vi "RSZVB Close.vi"(8 "error in (no error)":errorcluster {"code" format="%.0x"}, 11 "VISA session":refnum<visa-resource-name>) -> (0 "error out":errorcluster {"code" format="%.0x"})   [LabVIEW 2015]
doc: "This VI closes the I/O interface with the instrument."
uses:
  _utility/RSZVB Global Data.vi
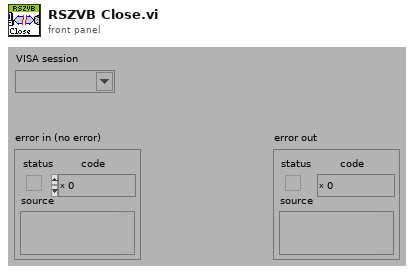
[diagram p1: front panel]
types:
  T1 = cluster{"Error Checking (T: On)":bool, "Installed Options":string[], "Data Valid?":bool, "Ports":i32, "Model":string[], "Option Checking (T: On)":bool}[]
  T2 = cluster{"Error Checking (T: On)":bool, "Installed Options":string[], "Data Valid?":bool, "Ports":i32, "Model":string[], "Option Checking (T: On)":bool}
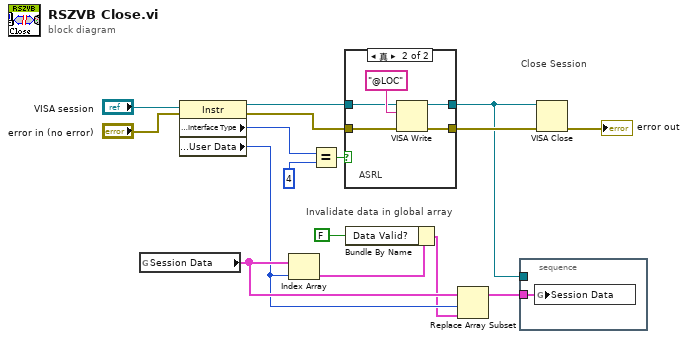
[diagram p0: block diagram]
diagram:
  # "Invalidate data in global array"
  # "Close Session"
  n1 = global read "RSZVB Global Data.vi" "Session Data"() -> (w7:T1)
  n2 = property class="Instr"(reference="VISA session", error in="error in (no error)") -> (reference out=w15:refnum<visa-resource-name>, error out=w14:errorcluster, "Interface Information:Interface Type"=w10:u16, "General Settings:User Data"=w4:u32)
  n3 = Index Array(array=w7, index=w4) -> (element=w6:T2)
  n4 = Equal?(x=w10, y=u16 4) -> (x = y?=w12:bool)
  n5 = case shown="真" w12 {
    tunnel: [w18 w22] -> w1
    tunnel: [w17 w21] -> w11
    tunnel: w15 -> [w18 w20]
    tunnel: w14 -> [w17 w19]
    frame False {
      # "GPIB"
    }
    frame True {
      # "ASRL"
      n6 = VISA Write(VISA resource name=w20, write buffer="@LOC" ("write buffer (\"\")"), error in (no error)=w19) -> (VISA resource name out=w22:refnum<visa-resource-name>, error out=w21:errorcluster)  [unwired: 1 out]
    }
  }
  n7 = Bundle By Name(cluster=w6, "Data Valid?"=FALSE) -> (w3:T2)
  n8 = Replace Array Subset(array=w7, new element=w3, index=w4) -> (w2:T1)
  n9 = stacked-sequence {
    tunnel: w2 -> [w24]
    tunnel: w1 -> [_]
    frame #0 {
      n10 = global write "RSZVB Global Data.vi" "Session Data"(w24) -> ()
    }
  }
  n11 = VISA Close(VISA resource name=w1, error in (no error)=w11) -> (error out=→"error out":errorcluster)
